vi "MICROWAVE Final.vi"() -> ()   [LabVIEW 2012]
panel:
  out "Timer (s)":dbl
  out "Pause":bool
  out "Opened Door":bool
  out "Rest":bool
  out "Timer (Count)":dbl
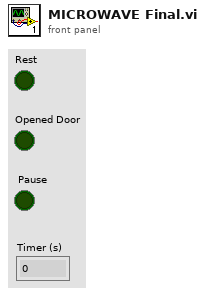
[diagram p1: front panel]
types:
  T1 = enum16{"Heating", "Rest", "Pause", "Opened Door", "Buzzer Beep"}
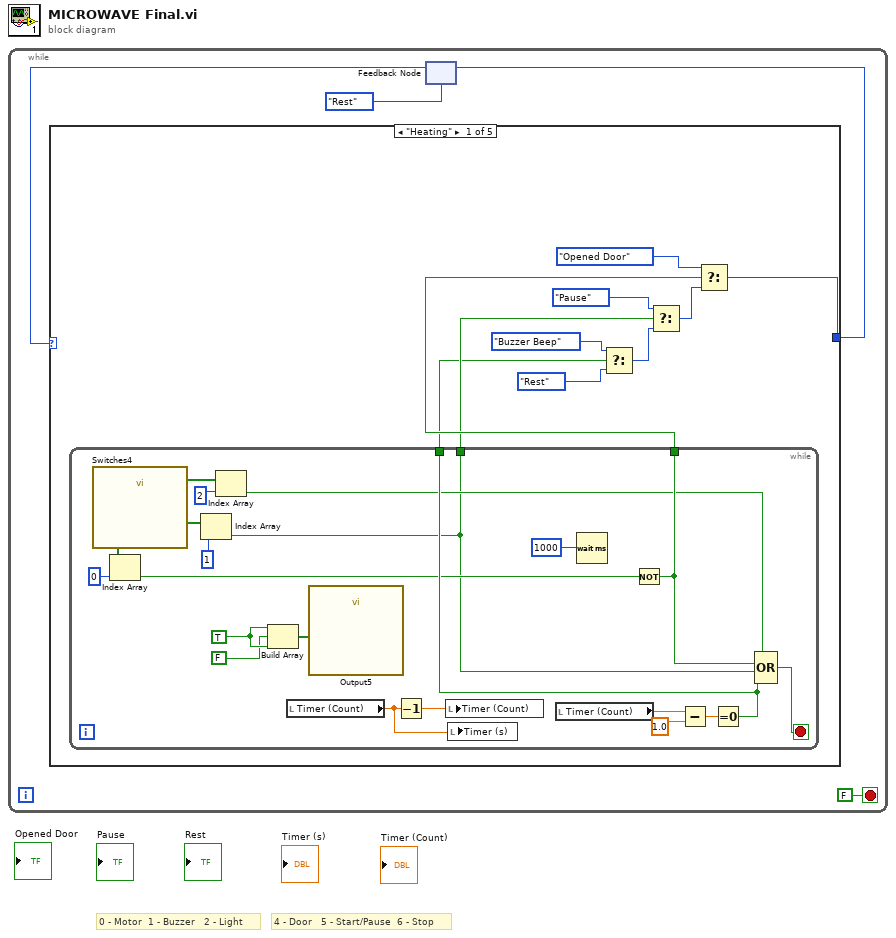
[diagram p0: block diagram]
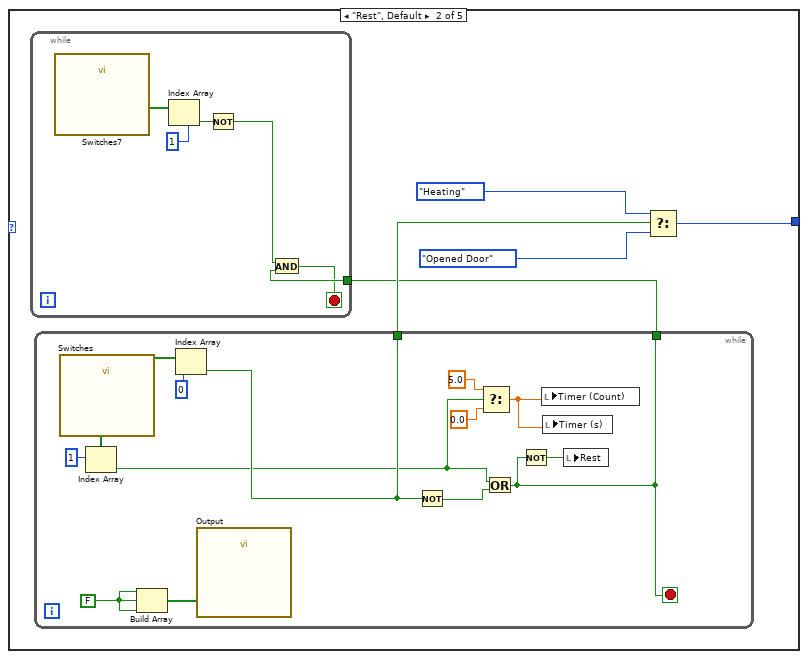
[diagram p2: hidden frame]
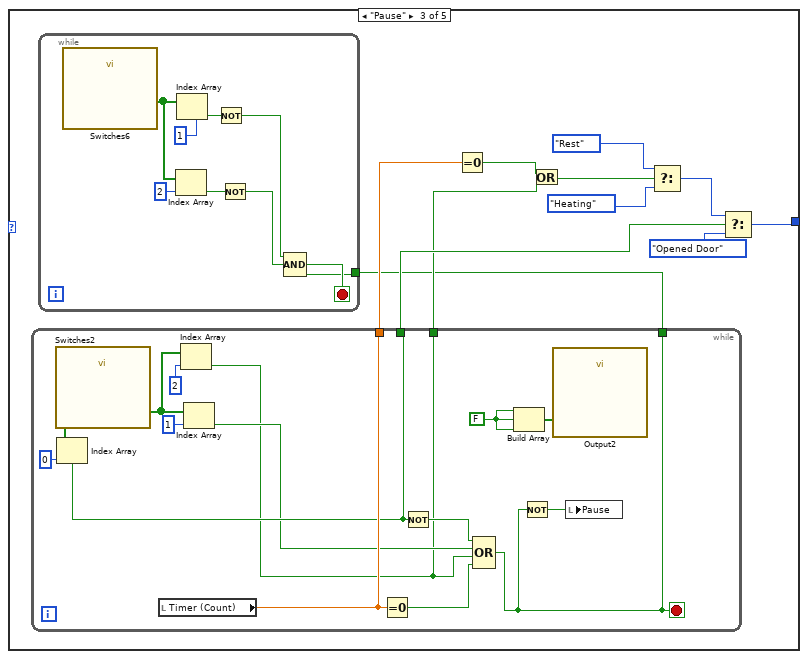
[diagram p3: hidden frame]
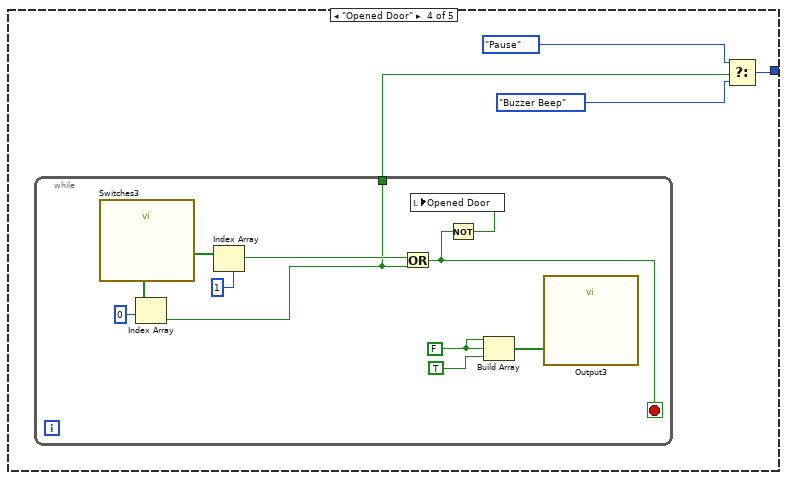
[diagram p4: hidden frame]
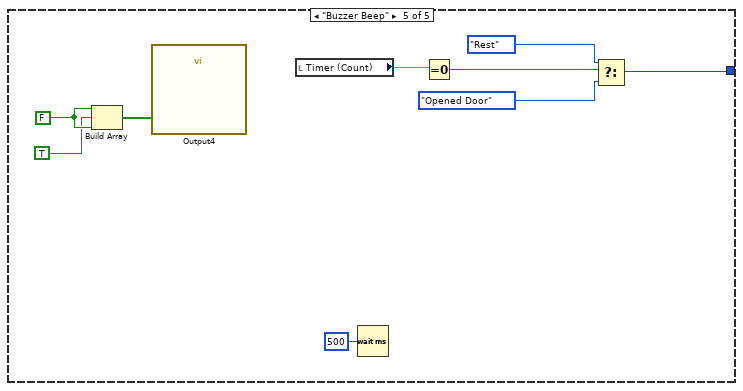
[diagram p5: hidden frame]
diagram:
  # "4 - Door   5 - Start/Pause  6 - Stop"
  # "0 - Motor  1 - Buzzer   2 - Light"
  n1 = while {
    stop <- FALSE stop-if-true
    n2 = feedback #1(T1."Rest") -> (w2:T1)
    n3 = case shown="\"Heating\"" w2 {
      tunnel: [w14 w38 w65 w95 w113] -> w3
      frame "Heating" {
        n4 = while {
          tunnel: [w32] -> w10
          tunnel: [w16] -> w9
          tunnel: [w26] -> w6
          stop <- w15 stop-if-true
          w25 = TRUE
          n5 = call "Switches4"() -> ("data"=w20:bool[])  [unwired: 17 in, 2 out]
          n6 = Index Array(array=w20, index=0) -> (element=w18:bool)
          n7 = Index Array(array=w20, index=1) -> (element=w16:bool)
          n8 = Index Array(array=w20, index=2) -> (element=w17:bool)
          n9 = Build Array(w25, FALSE ("element"), w25) -> (w24:bool[])
          n10 = local read "Timer (Count)"() -> (w27:dbl)
          n11 = call "Output5"("data"=w24) -> ()  [unwired: 17 in, 2 out]
          n12 = Decrement(x=w27) -> (x-1=w28:dbl)
          n13 = local write "Timer (Count)"(w28) -> ()
          n14 = local write "Timer (s)"(w27) -> ()
          n15 = local read "Timer (Count)"() -> (w31:dbl)
          n16 = Wait (ms)(milliseconds to wait=u32 1000 ("millisecond timer value")) -> ()  [unwired: 1 out]
          n17 = Not(x=w18) -> (.not. x?=w32:bool)
          n18 = Subtract(x=w31, y=1.0) -> (x-y=w30:dbl)
          n19 = Equal To 0?(x=w30) -> (x = 0?=w26:bool)
          n20 = Compound Arithmetic op=OR(w17, w32, w16, w26) -> (w15:bool)
        }
        n21 = Select(t=T1."Buzzer Beep", s=w6, f=T1."Rest") -> (s? t:f=w8:T1)
        n22 = Select(t=T1."Pause", s=w9, f=w8) -> (s? t:f=w12:T1)
        n23 = Select(t=T1."Opened Door", s=w10, f=w12) -> (s? t:f=w14:T1)
      }
      frame "Rest", Default {
        n24 = while {
          tunnel: [w47] -> w35
          tunnel: [w45] -> w34
          stop <- w45 stop-if-true
          w49 = FALSE
          n25 = call "Switches"() -> ("data"=w52:bool[])  [unwired: 17 in, 2 out]
          n26 = Index Array(array=w52, index=1) -> (element=w46:bool)
          n27 = Build Array(w49, w49, w49) -> (w48:bool[])
          n28 = Index Array(array=w52, index=0) -> (element=w47:bool)
          n29 = call "Output"("data"=w48) -> ()  [unwired: 17 in, 2 out]
          n30 = Not(x=w47) -> (.not. x?=w50:bool)
          n31 = Select(t=5.0, s=w46, f=0.0 ("t")) -> (s? t:f=w54:dbl)
          n32 = Or(x=w46, y=w50) -> (x .or. y?=w45:bool)
          n33 = Not(x=w45) -> (.not. x?=w57:bool)
          n34 = local write "Timer (Count)"(w54) -> ()
          n35 = local write "Timer (s)"(w54) -> ()
          n36 = local write "Rest"(w57) -> ()
        }
        n37 = while {
          tunnel: w34 -> [w41]
          stop <- w40 stop-if-true
          n38 = call "Switches7"() -> ("data"=w44:bool[])  [unwired: 17 in, 2 out]
          n39 = Index Array(array=w44, index=1) -> (element=w42:bool)
          n40 = Not(x=w42) -> (.not. x?=w39:bool)
          n41 = And(x=w39, y=w41) -> (x .and. y?=w40:bool)
        }
        n42 = Select(t=T1."Heating", s=w35, f=T1."Opened Door") -> (s? t:f=w38:T1)
      }
      frame "Pause" {
        n43 = while {
          tunnel: [w81] -> w61
          tunnel: [w88] -> w59
          tunnel: [w79] -> w60
          tunnel: [w78] -> w58
          stop <- w78 stop-if-true
          w87 = FALSE
          n44 = call "Switches2"() -> ("data"=w83:bool[])  [unwired: 17 in, 2 out]
          n45 = Index Array(array=w83, index=0) -> (element=w81:bool)
          n46 = local read "Timer (Count)"() -> (w88:dbl)
          n47 = Index Array(array=w83, index=2) -> (element=w79:bool)
          n48 = Index Array(array=w83, index=1) -> (element=w80:bool)
          n49 = Equal To 0?(x=w88) -> (x = 0?=w89:bool)
          n50 = Not(x=w81) -> (.not. x?=w90:bool)
          n51 = Compound Arithmetic op=OR(w90, w80, w79, w89) -> (w78:bool)
          n52 = Build Array(w87, w87, w87) -> (w86:bool[])
          n53 = Not(x=w78) -> (.not. x?=w91:bool)
          n54 = call "Output2"("data"=w86) -> ()  [unwired: 17 in, 2 out]
          n55 = local write "Pause"(w91) -> ()
        }
        n56 = while {
          tunnel: w58 -> [w69]
          stop <- w75 stop-if-true
          n57 = call "Switches6"() -> ("data"=w72:bool[])  [unwired: 17 in, 2 out]
          n58 = Index Array(array=w72, index=2) -> (element=w71:bool)
          n59 = Index Array(array=w72, index=1) -> (element=w76:bool)
          n60 = Not(x=w76) -> (.not. x?=w74:bool)
          n61 = Not(x=w71) -> (.not. x?=w70:bool)
          n62 = Compound Arithmetic op=AND(w74, w70, w69) -> (w75:bool)
        }
        n63 = Equal To 0?(x=w59) -> (x = 0?=w66:bool)
        n64 = Or(x=w66, y=w60) -> (x .or. y?=w63:bool)
        n65 = Select(t=T1."Rest", s=w63, f=T1."Heating") -> (s? t:f=w64:T1)
        n66 = Select(t=w64, s=w61, f=T1."Opened Door") -> (s? t:f=w65:T1)
      }
      frame "Opened Door" {
        n67 = while {
          tunnel: [w97] -> w92
          stop <- w96 stop-if-true
          w104 = FALSE
          n68 = call "Switches3"() -> ("data"=w101:bool[])  [unwired: 17 in, 2 out]
          n69 = Index Array(array=w101, index=0) -> (element=w97:bool)
          n70 = Index Array(array=w101, index=1) -> (element=w98:bool)
          n71 = Or(x=w98, y=w97) -> (x .or. y?=w96:bool)
          n72 = Not(x=w96) -> (.not. x?=w105:bool)
          n73 = local write "Opened Door"(w105) -> ()
          n74 = Build Array(w104, w104, TRUE ("element")) -> (w103:bool[])
          n75 = call "Output3"("data"=w103) -> ()  [unwired: 17 in, 2 out]
        }
        n76 = Select(t=T1."Pause", s=w92, f=T1."Buzzer Beep") -> (s? t:f=w95:T1)
      }
      frame "Buzzer Beep" {
        w108 = FALSE
        n77 = Build Array(w108, TRUE ("element"), w108) -> (w107:bool[])
        n78 = call "Output4"("data"=w107) -> ()  [unwired: 17 in, 2 out]
        n79 = local read "Timer (Count)"() -> (w109:dbl)
        n80 = Wait (ms)(milliseconds to wait=u32 500) -> ()  [unwired: 1 out]
        n81 = Equal To 0?(x=w109) -> (x = 0?=w112:bool)
        n82 = Select(t=T1."Rest", s=w112, f=T1."Opened Door") -> (s? t:f=w113:T1)
      }
    }
    n83 = feedback-in #1(w3) -> ()
  }
